vi "Route Specification from Listbox.vi"(8 "error in (no error)":errorcluster, 11 "listbox reference":refnum<vi>) -> (0 "error out":errorcluster, 1 "route specification":string, 2 "Indices of Routes":i32[](array[numeric]), 3 "listbox reference out":refnum<vi>)   [LabVIEW 2023, in "SwitchExecController.lvlib"]
uses:
  SwitchExecController.lvlib
  <vilib>/Utility/error.llb/Trim Whitespace One-Sided.vi
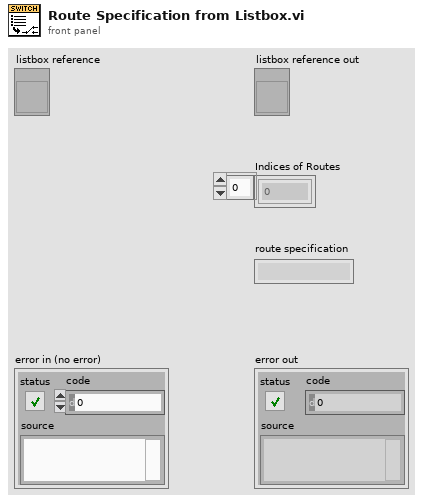
[diagram p1: front panel]
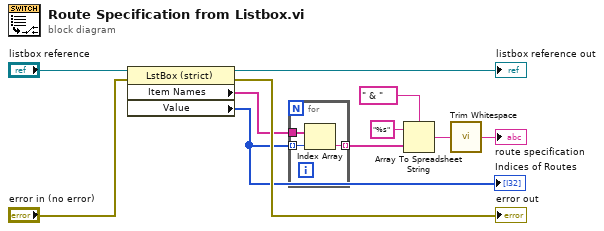
[diagram p0: block diagram]
diagram:
  n1 = property on="Property Node" class="LstBox (strict)"(reference="listbox reference", error in="error in (no error)") -> (reference out=→"listbox reference out":refnum<vi>, error out=→"error out":errorcluster, "Item Names"=w8:string[], "Value"=w9:i32[])
  "Indices of Routes" <- w9
  n2 = for {
    tunnel: w9 -> [w13] mode=indexing
    tunnel: w8 -> [w14]
    tunnel: [w12] -> w7 mode=indexing
    n3 = Index Array(array=w14, index=w13) -> (element=w12:string)
  }
  n4 = Array To Spreadsheet String(delimiter (Tab)=" & ", array=w7, 3:"%s" ("format string")) -> (spreadsheet string=w5:string)
  n5 = call <vilib>:"Trim Whitespace.vi"("string"=w5) -> ("trimmed string"=→"route specification":string)  [unwired: 1 in]
